vi "PusherServo Set Position.vi"(8 "Error":errorcluster, 9 "Stroke (0-100)":dbl, 11 "ServoDeviceRef":T1) -> (0 "Error Out":errorcluster, 2 "Stroke Set":dbl, 3 "ServoDeviceRef Out":T1)   [LabVIEW 2023, in "Feeder_ACT.lvlib"]
uses:
  Feeder_ACT.lvlib
  <vilib>/Rock Robotics/WPI/PWM/Servo/WPI_ServoDeviceRef.ctl
  <vilib>/Rock Robotics/SystemInterfaces/DIO/FPGA_DIOPWMChannel.ctl
  <vilib>/Rock Robotics/WPI/PWM/WPI_PWMDeadband.ctl
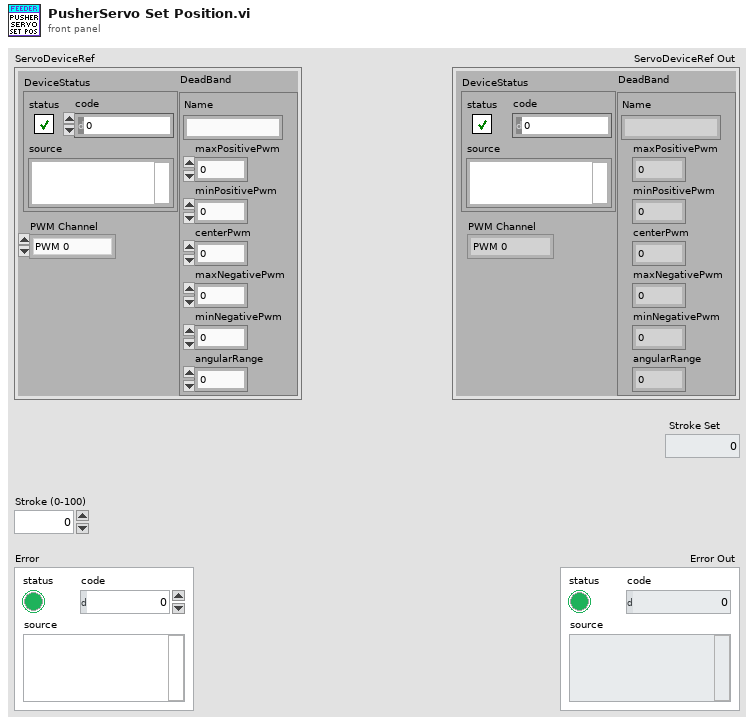
[diagram p1: front panel]
types:
  T1 = typedef "WPI_ServoDeviceRef.ctl" = cluster{"DeviceStatus":errorcluster, "PWM Channel":T2, "DeadBand":T3}
  T2 = typedef "FPGA_DIOPWMChannel.ctl" = enum8{"PWM 0", "PWM 1", "PWM 2", "PWM 3", "PWM 4", "PWM 5", "PWM 6", "PWM 7", "PWM 8", "PWM 9", "PWM MXP 0", "PWM MXP 1", "PWM MXP 2", "PWM MXP 3", "PWM MXP 4", "PWM MXP 5", "PWM MXP 6", "PWM MXP 7", "PWM MXP 8", "PWM MXP 9", "Invalid"}
  T3 = typedef "WPI_PWMDeadband.ctl" = cluster{"Name":string, "maxPositivePwm":i32, "minPositivePwm":i32, "centerPwm":i32, "maxNegativePwm":i32, "minNegativePwm":i32, "angularRange":u16}
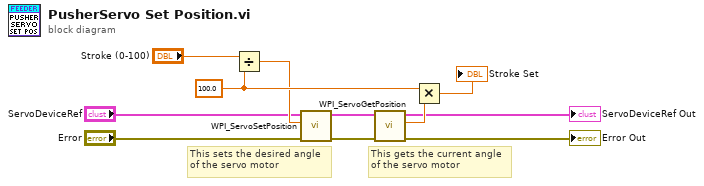
[diagram p0: block diagram]
diagram:
  w11 = 100.0 ("y")
  # "This gets the current angle\nof the servo motor"
  # "This sets the desired angle \nof the servo motor"
  n1 = Divide(x="Stroke (0-100)", y=w11) -> (x/y=w8:dbl)
  n2 = call <vilib>:"WPI_ServoSetPosition.vi"("error in (no error)"="Error", "Position"=w8, "ServoDeviceRef"="ServoDeviceRef") -> ("error out"=w2:errorcluster, "ServoDeviceRef"=w6:T1)  [unwired: 7 out]
  n3 = call <vilib>:"WPI_ServoGetPosition.vi"("error in (no error)"=w2, "ServoDeviceRef"=w6) -> ("error out"=→"Error Out":errorcluster, "Position"=w9:dbl, "ServoDeviceRef"=→"ServoDeviceRef Out":T1)  [unwired: 7 out]
  n4 = Multiply(x=w11, y=w9) -> (x*y=→"Stroke Set":dbl)
